vi "Util_Progress Progress Popup.vi"(10 "Message":string) -> ()   [LabVIEW 2013]
uses:
  FP Control/FP Control Functions.ctl
panel:
  in  "Stop":bool
  out "Message out":string
  out "Progress":i32(slide) scale=0.0..100.0
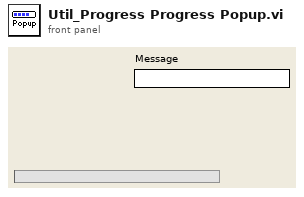
[diagram p1: front panel]
types:
  T1 = typedef "FP Control Functions.ctl" = enum16{"Open", "Close", "Bring To Front", "Center"}
  T2 = cluster{"left":i16, "top":i16, "right":i16, "bottom":i16}
  T3 = typedef "LVRectTypeDef.ctl" = cluster{"Left":i16, "Top":i16, "Right":i16, "Bottom":i16}
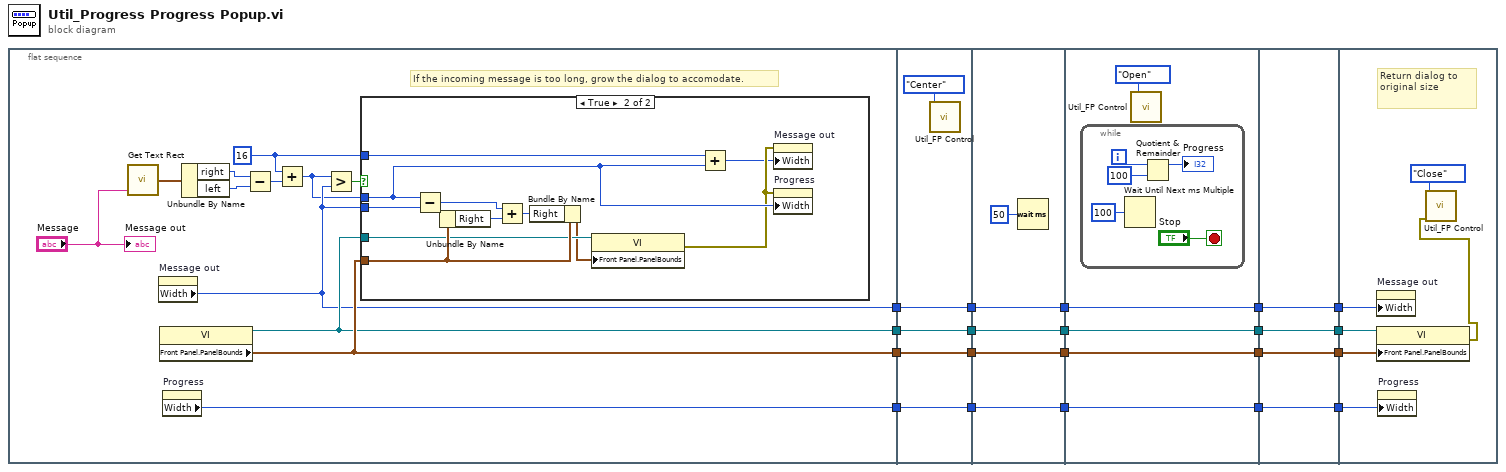
[diagram p0: block diagram]
diagram:
  n1 = flat-sequence {
    tunnel: [w25] -> w18
    tunnel: [w27] -> w15
    tunnel: [w28] -> w12
    tunnel: [w29] -> w9
    tunnel: [w48] -> w8
    tunnel: w18 -> [w48]
    tunnel: [w47] -> w6
    tunnel: w15 -> [w47]
    tunnel: [w46] -> w4
    tunnel: w12 -> [w46]
    tunnel: [w45] -> w2
    tunnel: w9 -> [w45]
    tunnel: w8 -> [w53]
    tunnel: [w53] -> w7
    tunnel: w6 -> [w52]
    tunnel: [w52] -> w5
    tunnel: w4 -> [w51]
    tunnel: [w51] -> w3
    tunnel: w2 -> [w50]
    tunnel: [w50] -> w1
    tunnel: [w58] -> w19
    tunnel: w7 -> [w58]
    tunnel: [w57] -> w16
    tunnel: w5 -> [w57]
    tunnel: [w56] -> w13
    tunnel: w3 -> [w56]
    tunnel: [w55] -> w10
    tunnel: w1 -> [w55]
    tunnel: [w67] -> w20
    tunnel: w19 -> [w67]
    tunnel: [w66] -> w17
    tunnel: w16 -> [w66]
    tunnel: [w65] -> w14
    tunnel: w13 -> [w65]
    tunnel: [w64] -> w11
    tunnel: w10 -> [w64]
    tunnel: w20 -> [w73]
    tunnel: w17 -> [w72]
    tunnel: w14 -> [w71]
    tunnel: w11 -> [w70]
    frame #0 {
      w21 = i16 16 ("y")
      # "If the incoming message is too long, grow the dialog to accomodate."
      n2 = call <vilib>:"Get Text Rect.vi"("text"="Message") -> ("rect"=w32:T2)  [unwired: 8 in]
      n3 = property on="Message out" class="Str"() -> ("Width"=w25:u32)  [unwired: 2 in, 2 out]
      n4 = property class="VI"() -> (reference out=w27:refnum<vi>, "Front Panel.PanelBounds"=w28:T3)  [unwired: 2 in, 1 out]
      n5 = property on="Progress" class="Slide (strict)"() -> ("Width"=w29:u32)  [unwired: 2 in, 2 out]
      n6 = Unbundle By Name(w32) -> ("right"=w31:i16, "left"=w30:i16)
      n7 = Subtract(x=w31, y=w30) -> (x-y=w22:i16)
      n8 = Add(x=w21, y=w22) -> (x+y=w24:i16)
      n9 = Greater?(x=w24, y=w25) -> (0:w23:bool)
      n10 = case shown="True" w23 {
        tunnel: w24 -> [_ w43]
        tunnel: w28 -> [_ w42]
        tunnel: w27 -> [_ w41]
        tunnel: w25 -> [_ w40]
        tunnel: w21 -> [_ w33]
        frame False {
        }
        frame True {
          n11 = Subtract(x=w43, y=w40) -> (x-y=w35:u32)
          n12 = Unbundle By Name(w42) -> ("Right"=w36:i16)
          n13 = Add(x=w35, y=w36) -> (x+y=w39:u32)
          n14 = Bundle By Name(cluster=w42, "Right"=w39) -> (w38:T3)
          n15 = property class="VI"(reference=w41, "Front Panel.PanelBounds"=w38) -> (error out=w37:errorcluster)  [unwired: 1 in, 1 out]
          n16 = Add(x=w33, y=w43) -> (x+y=w34:i16)
          n17 = property on="Message out" class="Str"(error in=w37, "Width"=w34) -> ()  [unwired: 1 in, 2 out]
          n18 = property on="Progress" class="Slide (strict)"(error in=w37, "Width"=w43) -> ()  [unwired: 1 in, 2 out]
        }
      }
      "Message out" <- "Message"
    }
    frame #1 {
      n19 = call "Util_FP Control.vi"("Function"=FP_Control_Functions."Center") -> ()  [unwired: 1 in, 10 out]
    }
    frame #2 {
      n20 = Wait (ms)(milliseconds to wait=u32 50) -> ()  [unwired: 1 out]
    }
    frame #3 {
      n21 = while {
        i -> [w63]
        stop <- "Stop" stop-if-true
        n22 = Wait Until Next ms Multiple(millisecond multiple=u32 100) -> ()  [unwired: 1 out]
        n23 = Quotient & Remainder(x=w63, y=100) -> (x-y*floor(x/y)=→"Progress":i32)  [unwired: 1 out]
      }
      n24 = call "Util_FP Control.vi"("Function"=FP_Control_Functions."Open") -> ()  [unwired: 1 in, 10 out]
    }
    frame #4 {
    }
    frame #5 {
      # "Return dialog to original size"
      n25 = property on="Message out" class="Str"("Width"=w73) -> ()  [unwired: 2 in, 2 out]
      n26 = property class="VI"(reference=w72, "Front Panel.PanelBounds"=w71) -> (error out=w68:errorcluster)  [unwired: 1 in, 1 out]
      n27 = property on="Progress" class="Slide (strict)"("Width"=w70) -> ()  [unwired: 2 in, 2 out]
      n28 = call "Util_FP Control.vi"("error in (no error)"=w68, "Function"=FP_Control_Functions."Close") -> ()  [unwired: 10 out]
    }
  }
